vi "DigitalOutput-Daemon.vi"(3 "Configuration":T2={"Output Lines"=["BNC_Panel/port0/line1", "BNC_Panel/port0/line2", "BNC_Panel/port0/line3"], "DO timestamp lines"=["BNC_Panel/port0/line0", "BNC_Panel/port0/line0", "BNC_Panel/port0/line0"], "Timestamp lines"=["BNC_Panel/port0/line0"]}, 4 "OutputRequest\nuser event refnum":T1) -> ()   [LabVIEW 2011]
doc: "OutputRequest handler for the DigitalOutput output device. \n\nThis VI is meant to be started asynchronously. It will register itself as a listener on the OutputRequest user event refnum and process any requests that it knows how to handle.\n\nThe \"Configuration\" structure is used for initialization and contains:\n\"Timestamp Line\": Device address for timestamp line\n\"Output Lines\": Array of device addresses for digital output\n\nCommands handled by this VI:\nTarget = \"all\"\n stop: Unregisters and stops running.\nTarget = \"digitalOutput\"\n switch;[index];[\"on\"/\"off\"]; switches that port on (high) or off (low)\n pulse;[index];[\"on\"/\"off\"];[length]; pulses for the specified length (ms)\nTarget = \"timestampedDigitalOutput\"\n [message];[restOfCommand] pulses TS line, incr. TS count, executes rest of command\nTarget = \"timestamp\" or \"timestamped*\" (except AnalogOutput)\n pulses TS line and increments the TS count"
uses:
  DigitalOutput-Configuration.ctl
  Typedefs/OutputRequest refnum.ctl
  Typedefs/OutputRequest.ctl
panel:
  out "TS only":refnum<k21>[](array[refnum])
  out "line+TS":refnum<k21>[](array[refnum])
  out "line only":refnum<k21>[](array[refnum])
  # "Digital output tasks"
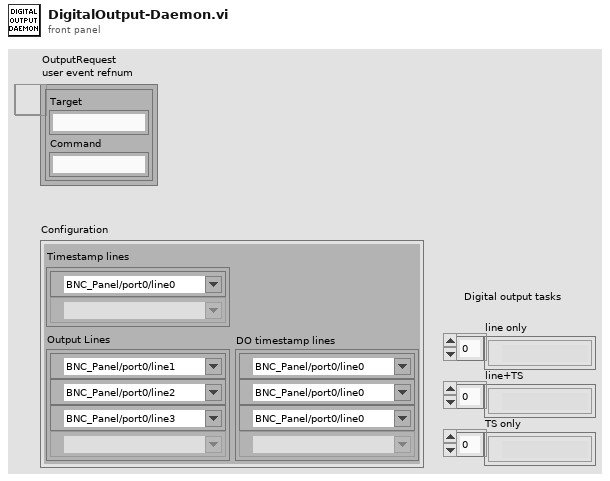
[diagram p1: front panel]
types:
  T1 = typedef "OutputRequest refnum.ctl" = refnum<user-event>
  T2 = typedef "DigitalOutput-Configuration.ctl" = cluster{"Output Lines":tag[], "DO timestamp lines":tag[], "Timestamp lines":tag[]}
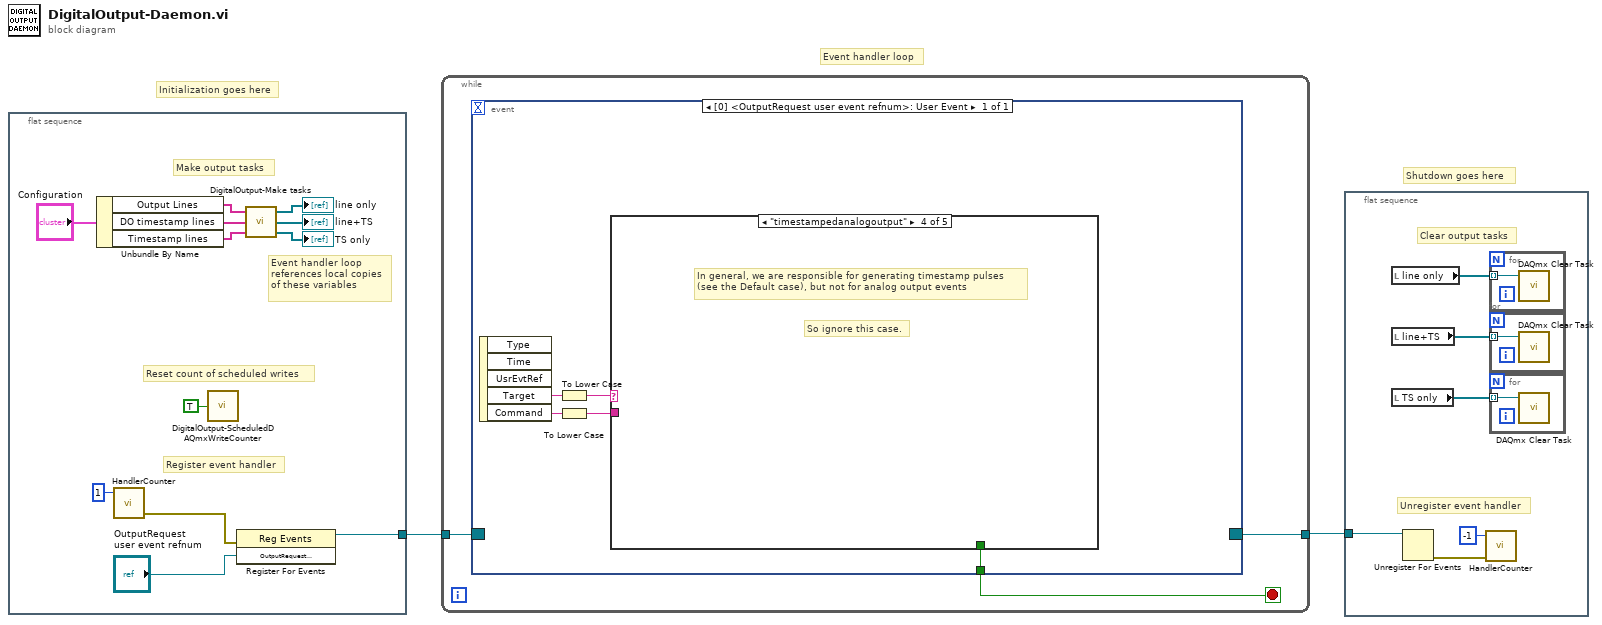
[diagram p0: block diagram]
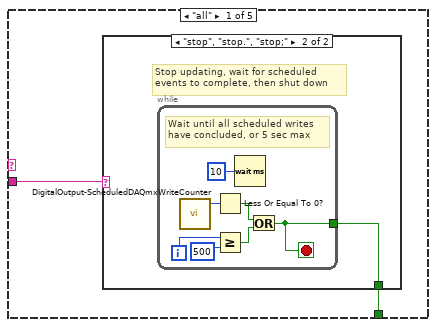
[diagram p2: hidden frame]
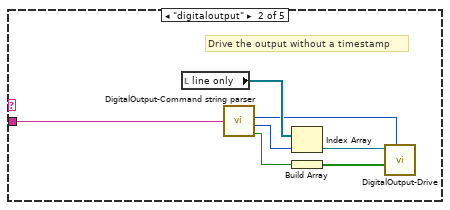
[diagram p4: hidden frame]
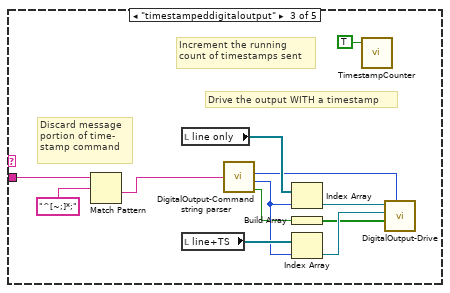
[diagram p5: hidden frame]
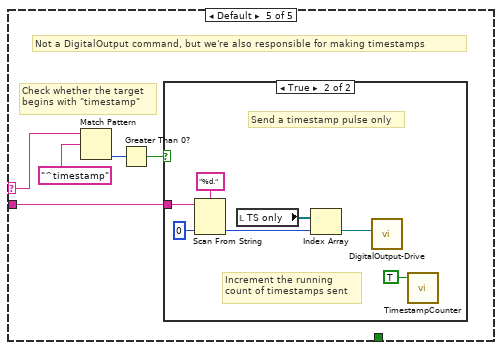
[diagram p6: hidden frame]
diagram:
  # "Shutdown goes here"
  # "Event handler loop"
  # "Initialization goes here"
  n1 = flat-sequence {
    tunnel: [w14] -> w2
    frame #0 {
      # "Reset count of scheduled writes"
      # "Event handler loop\nreferences local copies\nof these variables"
      # "Make output tasks"
      # "Register event handler"
      n2 = Unbundle By Name("Configuration") -> ("Output Lines"=w6:tag[], "DO timestamp lines"=w8:tag[], "Timestamp lines"=w4:tag[])
      n3 = call "HandlerCounter.vi"("Change in count"=i16 1) -> ("error out"=w13:errorcluster)  [unwired: 3 in, 1 out]
      n4 = call "DigitalOutput-ScheduledDAQmxWriteCounter.vi"("Reset Count"=TRUE) -> ()  [unwired: 3 in, 2 out]
      n5 = register-events(error in=w13, "OutputRequest\nuser event refnum") -> (reference out=w14:refnum<event-registration>)  [unwired: 1 in, 1 out]
      n6 = call "DigitalOutput-Make tasks.vi"("Timestamp lines"=w4, "DO timestamp lines"=w8, "Output Lines"=w6) -> ("TS only"=→"TS only":refnum<k21>[], "line+TS"=→"line+TS":refnum<k21>[], "line only"=→"line only":refnum<k21>[])
    }
  }
  n7 = while {
    tunnel: w2 -> [w17]
    tunnel: [w16] -> w1
    stop <- w15 stop-if-true
    n8 = event shown="[0] <OutputRequest\nuser event refnum>: User Event" {
      selector: w17 -> [_]
      dyn-events: [_] -> w16
      timeout: _ -> [_]
      tunnel: [w22] -> w15
      event User Event {
        n9 = event-data() -> ("Target"=w21:string, "Command"=w19:string)  [unwired: 1 in, 3 out]
        n10 = To Lower Case(string=w21) -> (all lower case string=w20:string)
        n11 = To Lower Case(string=w19) -> (all lower case string=w18:string)
        n12 = case shown="\"timestampedanalogoutput\"" w20 {
          selector: w20 -> [_ _ _ _ w55]
          tunnel: w18 -> [w24 w33 w48 _ w52]
          tunnel: [w23 _ _ _ _] -> w22
          frame "all" {
            n13 = case shown="\"stop\", \"stop.\", \"stop;\"" w24 {
              tunnel: [_ w25] -> w23
              frame Default {
                # "Unrecognized command.\nWe should probably put some\nerror throwing code here..."
              }
              frame "stop", "stop.", "stop;" {
                # "Stop updating, wait for scheduled\nevents to complete, then shut down"
                n14 = while {
                  tunnel: [w26] -> w25
                  i -> [w30]
                  stop <- w26 stop-if-true
                  # "Wait until all scheduled writes \nhave concluded, or 5 sec max"
                  n15 = call "DigitalOutput-ScheduledDAQmxWriteCounter.vi"() -> ("Count"=w31:i16)  [unwired: 4 in, 1 out]
                  n16 = Less Or Equal To 0?(x=w31) -> (x <= 0?=w27:bool)
                  n17 = Greater Or Equal?(x=w30, y=500) -> (x >= y?=w28:bool)
                  n18 = Wait (ms)(milliseconds to wait=u32 10) -> ()  [unwired: 1 out]
                  n19 = Or(x=w27, y=w28) -> (x .or. y?=w26:bool)
                }
              }
            }
          }
          frame "digitaloutput" {
            # "Drive the output without a timestamp"
            n20 = local read "line only"() -> (w39:refnum<k21>[])
            n21 = call "DigitalOutput-Command string parser.vi"("Command string"=w33) -> ("Pulse length (ms)"=w37:i32, "Line index"=w38:i32, "Drive high?"=w34:bool)  [unwired: 1 in]
            n22 = Index Array(array=w39, index=w38) -> (element=w36:refnum<k21>)
            n23 = Build Array(w34) -> (w35:bool[])
            n24 = call "DigitalOutput-Drive.vi"("duration (-1 = cont.)"=w37, "data"=w35, "line only"=w36) -> ()  [unwired: 8 in, 1 out]
          }
          frame "timestampeddigitaloutput" {
            # "Discard message\nportion of time-\nstamp command"
            # "Increment the running\ncount of timestamps sent"
            # "Drive the output WITH a timestamp"
            n25 = Match Pattern(string=w48, regular expression="^[~;]*;") -> (after substring=w49:string)  [unwired: 1 in, 3 out]
            n26 = local read "line only"() -> (w51:refnum<k21>[])
            n27 = local read "line+TS"() -> (w46:refnum<k21>[])
            n28 = call "DigitalOutput-Command string parser.vi"("Command string"=w49) -> ("Pulse length (ms)"=w44:i32, "Line index"=w45:i32, "Drive high?"=w40:bool)  [unwired: 1 in]
            n29 = Index Array(array=w51, index=w45) -> (element=w42:refnum<k21>)
            n30 = Build Array(w40) -> (w41:bool[])
            n31 = Index Array(array=w46, index=w45) -> (element=w43:refnum<k21>)
            n32 = call "TimestampCounter.vi"("Increment"=TRUE) -> ()  [unwired: 3 in, 2 out]
            n33 = call "DigitalOutput-Drive.vi"("duration (-1 = cont.)"=w44, "data"=w41, "line+TS"=w43, "line only"=w42) -> ()  [unwired: 7 in, 1 out]
          }
          frame "timestampedanalogoutput" {
            # "So ignore this case."
            # "In general, we are responsible for generating timestamp pulses\n(see the Default case), but not for analog output events"
          }
          frame Default {
            # "Not a DigitalOutput command, but we're also responsible for making timestamps"
            # "Check whether the target\nbegins with \"timestamp\""
            n34 = Match Pattern(string=w55, regular expression="^timestamp") -> (offset past match=w54:i32)  [unwired: 1 in, 3 out]
            n35 = Greater Than 0?(x=w54) -> (x > 0?=w53:bool)
            n36 = case shown="True" w53 {
              tunnel: w52 -> [_ w62]
              frame False {
                # "Ignore the request, it doesn't pertain\nto this output device"
              }
              frame True {
                # "Increment the running\ncount of timestamps sent"
                # "Send a timestamp pulse only"
                n37 = Scan From String(format string="%d.", input string=w62, default 1=0 ("default value 1")) -> (output 1=w59:i32)  [unwired: 2 in, 3 out]
                n38 = local read "TS only"() -> (w58:refnum<k21>[])
                n39 = Index Array(array=w58, index=w59) -> (element=w57:refnum<k21>)
                n40 = call "DigitalOutput-Drive.vi"("line+TS"=w57) -> ()  [unwired: 10 in, 1 out]
                n41 = call "TimestampCounter.vi"("Increment"=TRUE) -> ()  [unwired: 3 in, 2 out]
              }
            }
          }
        }
      }
    }
  }
  n42 = flat-sequence {
    tunnel: w1 -> [w69]
    frame #0 {
      # "Clear output tasks"
      # "Unregister event handler"
      n43 = local read "line only"() -> (w66:refnum<k21>[])
      n44 = local read "line+TS"() -> (w65:refnum<k21>[])
      n45 = local read "TS only"() -> (w64:refnum<k21>[])
      n46 = Unregister For Events(event registration refnum=w69) -> (error out=w68:errorcluster)  [unwired: 1 in]
      n47 = call "HandlerCounter.vi"("error in"=w68, "Change in count"=i16 -1) -> ()  [unwired: 2 in, 2 out]
      n48 = for {
        tunnel: w66 -> [w72] mode=indexing
        n49 = call <vilib>:"DAQmx Clear Task.vi"("task in"=w72) -> ()  [unwired: 14 in, 1 out]
      }
      n50 = for {
        tunnel: w65 -> [w71] mode=indexing
        n51 = call <vilib>:"DAQmx Clear Task.vi"("task in"=w71) -> ()  [unwired: 14 in, 1 out]
      }
      n52 = for {
        tunnel: w64 -> [w70] mode=indexing
        n53 = call <vilib>:"DAQmx Clear Task.vi"("task in"=w70) -> ()  [unwired: 14 in, 1 out]
      }
    }
  }
